vi "ADS1115_READ_N_SAMPLE.vi"(6 "options_i2c_read":T1, 7 "N_Samples":u32, 8 "error in (no error)":errorcluster, 9 "Scale Value (mV)":dbl=2.0, 10 "I2C Slave Address (0)":u8, 11 "handle":u32) -> (0 "error out":errorcluster, 1 "mV":dbl[](array[numeric]), 2 "Sample/s":dbl, 3 "handle out":u32)   [LabVIEW 2017]
uses:
  libMPSSE.lvlib
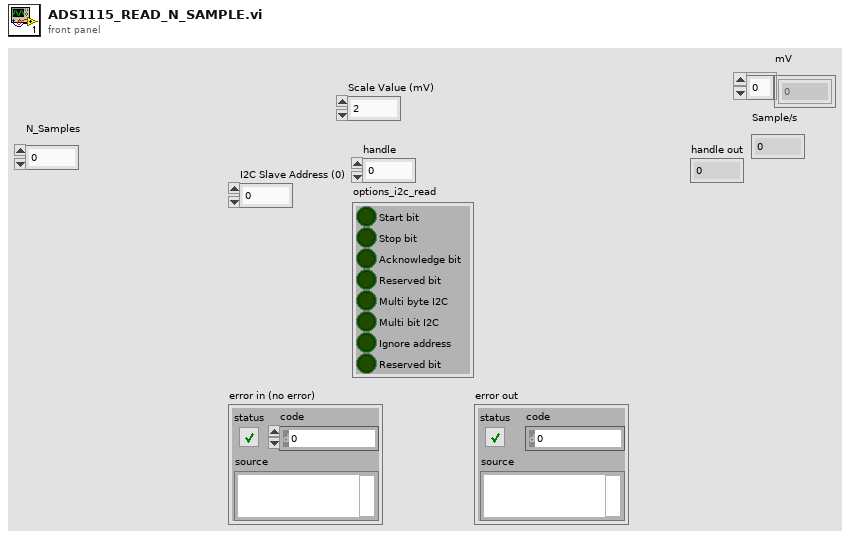
[diagram p1: front panel]
types:
  T1 = cluster{"Start bit":bool, "Stop bit":bool, "Acknowledge bit":bool, "Reserved bit":bool, "Multi byte I2C":bool, "Multi bit I2C":bool, "Ignore address":bool, "Reserved bit":bool}
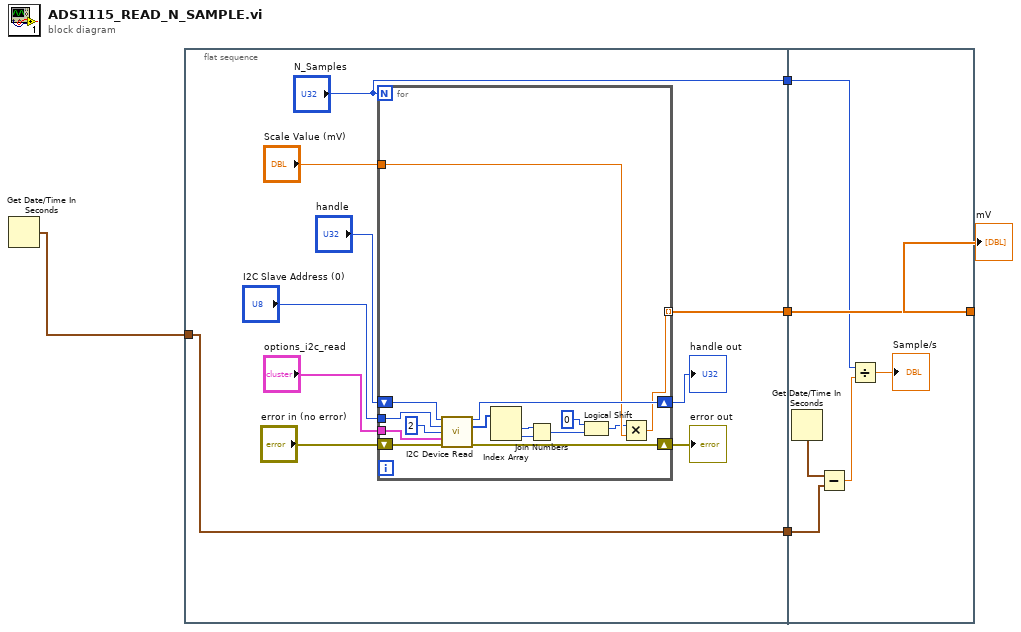
[diagram p0: block diagram]
diagram:
  n1 = Get Date/Time In Seconds() -> (seconds since 1Jan1904=w4:timestamp)
  n2 = flat-sequence {
    tunnel: w4 -> [w7]
    tunnel: [w8] -> w3
    tunnel: [w7] -> w2
    tunnel: ["N_Samples"] -> w1
    tunnel: [w36] -> w5
    tunnel: w3 -> [w36]
    tunnel: w2 -> [w34]
    tunnel: w1 -> [w33]
    frame #0 {
      n3 = for {
        N: "N_Samples" -> [_]
        tunnel: "I2C Slave Address (0)" -> [w29]
        tunnel: "options_i2c_read" -> [w24]
        tunnel: "Scale Value (mV)" -> [w23]
        shift-right: [w28] -> w13
        shift-left: "handle" -> [w30]
        shift-right: [w25] -> w11
        shift-left: "error in (no error)" -> [w26]
        tunnel: [w16] -> w8 mode=indexing
        n4 = call "I2C Device Read.vi"("handle"=w30, "Slave device address"=w29, "Size to transfer"=u32 2 ("Bytes To Read"), "options"=w24, "error in (no error)"=w26) -> ("handle out"=w28:u32, "Data read"=w27:u8[], "error out"=w25:errorcluster)  [unwired: 6 in, 2 out]
        n5 = Index Array(array=w27) -> (element #1=w20:u8, element #2=w21:u8)  [unwired: 2 in]
        n6 = Join Numbers(hi=w20, lo=w21) -> ((hi.lo)=w19:u16)
        n7 = Logical Shift(y=i8 0, x=w19) -> (x << y=w22:u16)
        n8 = Multiply(x=w22, y=w23) -> (x*y=w16:dbl)
      }
      "error out" <- w11
      "handle out" <- w13
    }
    frame #1 {
      n9 = Get Date/Time In Seconds() -> (seconds since 1Jan1904=w35:timestamp)
      n10 = Subtract(x=w35, y=w34) -> (x-y=w32:dbl)
      n11 = Divide(x=w33, y=w32) -> (x/y=→"Sample/s":dbl)
    }
  }
  "mV" <- w5
